vi "Deserialize JSON to LabVIEW Object.vi"() -> ()   [LabVIEW 2020]
doc: "This VI demonstrates a function of the GCraftsman JSON Serialization Toolkit.\n\nIt uses the 'Unflatten from JSON String' function to deserialize a JSON string into a LabVIEW object, including hierarchical and composite relationships.\n\nThis does not require the class to have accessor methods.\n\nGCraftsman JSON Object Serialization Toolkit\nwww.GCraftsman.com\nCopyright (c) 2017, GCraftsman"
uses:
  Class3/Class3.lvclass
  Class2/Class2.lvclass
  library/JKI JSON Object Serialization.lvlib
panel:
  out "myBool":bool
  out "anotherNumber":dbl format="%#_13g"
  out "someNumber":dbl format="%#_13g"
  out "myNum 2":dbl format="%#_13g"
  out "myNum":dbl format="%#_13g"
  out "unflattenedObj":refnum<class "Class2.lvclass">
  in  "JSON String":string="{\r\n    \"someNumber\":456,\r\n    \"myClass3Array\":[\r\n        {\r\n            \"myNum\":444\r\n        },\r\n        {\r\n            \"myNum\":555\r\n        }\r\n    ],\r\n    \"myBool\":true,\r\n    \"anotherNumber\":123\r\n}"
  # "This VI demonstrates a function of the GCraftsman JSON Serialization Toolkit.\n\nLook at the block diagram to see that the 'Unflatten from JSON String' function can deserialize a JSON string into a LabVIEW object, including hierarchical and composite relationships.\n\nRun this VI ."
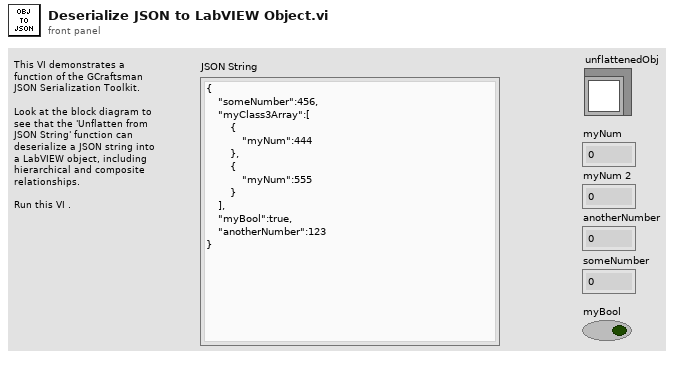
[diagram p1: front panel]
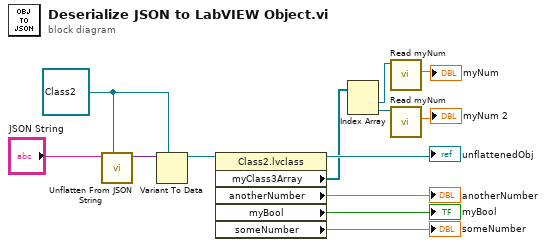
[diagram p0: block diagram]
diagram:
  w1 = refnum<class "Class2.lvclass"> refnum ("reference")
  n1 = call "Unflatten From JSON String.vi"("Type and Defaults"=w1, "JSON String"="JSON String") -> ("Variant"=w3:variant)  [unwired: 8 in, 1 out]
  n2 = Variant To Data(type=w1, Variant=w3) -> (data=w2:refnum<class "Class2.lvclass">)  [unwired: 1 in, 1 out]
  n3 = property class="Class2.lvclass"(reference=w2) -> (reference out=→"unflattenedObj":refnum<class "Class2.lvclass">, "myClass3Array"=w8:refnum<class "Class3.lvclass">[], "anotherNumber"=→"anotherNumber":dbl, "myBool"=→"myBool":bool, "someNumber"=→"someNumber":dbl)  [unwired: 1 in, 1 out]
  n4 = Index Array(array=w8) -> (element #1=w13:refnum<class "Class3.lvclass">, element #2=w12:refnum<class "Class3.lvclass">)  [unwired: 2 in]
  n5 = call "Read myNum.vi"("Class3 in"=w13) -> ("myNum"=→"myNum":dbl)  [unwired: 8 in, 2 out]
  n6 = call "Read myNum.vi"("Class3 in"=w12) -> ("myNum"=→"myNum 2":dbl)  [unwired: 8 in, 2 out]
